vi "Write Gain.vi"(8 "error in (no error)":errorcluster, 10 "Input Gain":dbl[](array[numeric]), 11 "Lockin.DAQ":refnum<class "Lockin.DAQ.lvclass">) -> (0 "error out":errorcluster, 3 "Lockin.DAQ out":refnum<class "Lockin.DAQ.lvclass">)   [LabVIEW 2016, in "Lockin.DAQ.lvclass"]
uses:
  Lockin.DAQ.lvclass
  Lockin.DAQ.lvclass/Lockin.DAQ.ctl
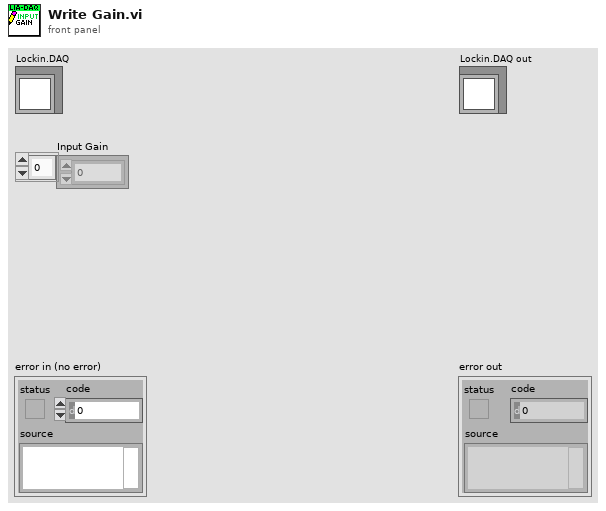
[diagram p1: front panel]
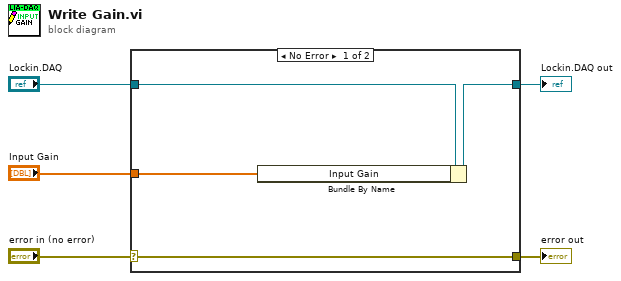
[diagram p0: block diagram]
diagram:
  n1 = case shown="No Error" "error in (no error)" {
    selector: "error in (no error)" -> [w9 w10]
    tunnel: [w9 w10] -> w4
    tunnel: [w7 w11] -> w2
    tunnel: "Lockin.DAQ" -> [w8 w11]
    tunnel: "Input Gain" -> [w6 _]
    frame No Error {
      n2 = Bundle By Name(cluster=w8, "Input Gain"=w6) -> (w7:refnum<class "Lockin.DAQ.lvclass">)
    }
    frame Error {
    }
  }
  "error out" <- w4
  "Lockin.DAQ out" <- w2
